vi "Menu_ItemName.vi"(7 "Ctrl":string, 8 "error in (no error)":errorcluster, 10 "DB Ref":T1, 11 "String":string) -> (0 "error out":errorcluster)   [LabVIEW 2017, in "tagdb-RefMgr Operations.lvlib"]
uses:
  tagdb-RefMgr Operations.lvlib
  <userlib>/_NEVSTOP/TagDB/Typedef/TagDB.ctl
  00d0da00-135c-4b50-b029-f1f1f0d03544.vi
  3fef5895-5f1b-4d45-a284-c279625095f7.vi
  4c542a80-f847-4821-836c-1c9f0a826a9d.vi
  00d0da00-135c-4b50-b029-f1f1f0d03544.vi/1b47866c-8e2d-43a7-815f-8cf18635e5a1.vi
  4c542a80-f847-4821-836c-1c9f0a826a9d.vi/1b47866c-8e2d-43a7-815f-8cf18635e5a1.vi
  <userlib>/_NEVSTOP/TagDB/_Support/Change Detector/TagDB dbChanged.vi
  <userlib>/_NEVSTOP/TagDB/_Support/Error/_Clear Errors.vi
  00d0da00-135c-4b50-b029-f1f1f0d03544.vi/1b47866c-8e2d-43a7-815f-8cf18635e5a1.vi/29b2ea6d-6d7f-4e4a-ad31-a5cb760462c7.vi
  <userlib>/_NEVSTOP/TagDB/API/TagDB-Status.vi
  4c542a80-f847-4821-836c-1c9f0a826a9d.vi/1b47866c-8e2d-43a7-815f-8cf18635e5a1.vi/29b2ea6d-6d7f-4e4a-ad31-a5cb760462c7.vi
  <userlib>/_NEVSTOP/TagDB/_Support/Change Detector/TagDB ChangeFlag.vi
  <userlib>/_NEVSTOP/TagDB/_Support/DataAccess/_NameCacher.vi
  <userlib>/_NEVSTOP/TagDB/_Support/Error/_[error50002]Invalid DataType.vi
  <userlib>/_NEVSTOP/TagDB/_Support/Error/_[error50000]Invalid DB REF.vi
  <userlib>/_NEVSTOP/TagDB/_Support/DataAccess/TagDB Ref to DVR.vi
  <userlib>/_NEVSTOP/TagDB/_Support/URL/TRIM-BOTH-SPACE.vi
  <userlib>/_NEVSTOP/TagDB/_Support/Error/_Build Error Cluster.vi
  <userlib>/_NEVSTOP/TagDB/TagDB.lvlib
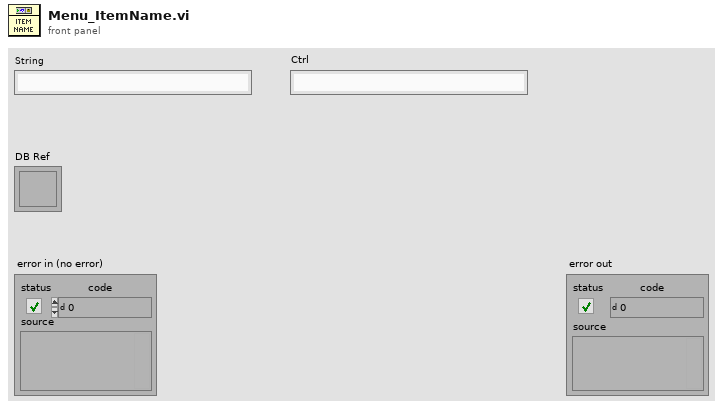
[diagram p1: front panel]
types:
  T1 = typedef "TagDB.lvlib/TagDB.ctl" = refnum<k1>
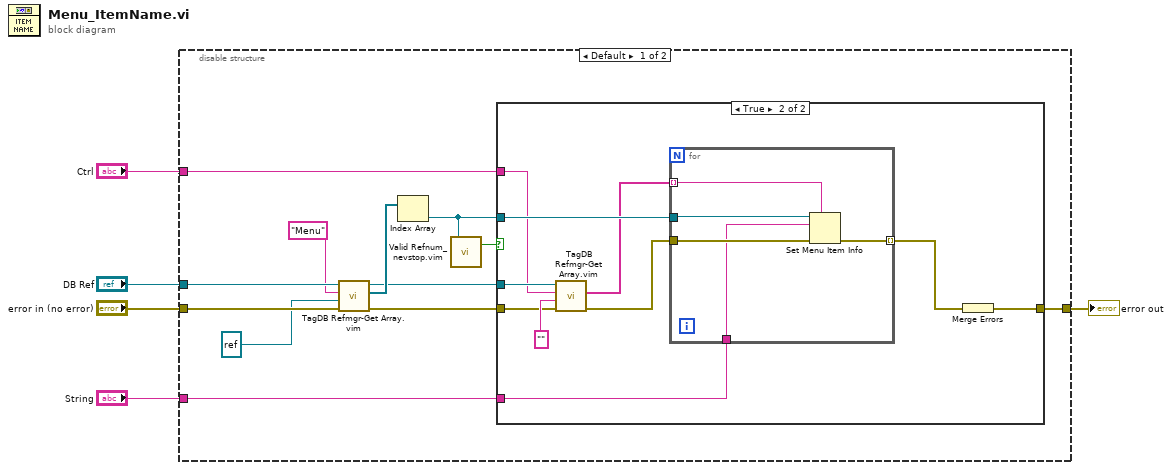
[diagram p0: block diagram]
diagram:
  n1 = disable-structure shown="Default" {
    disable-tunnel: "error in (no error)" -> [w17 w34]
    disable-tunnel: "DB Ref" -> [w16 _]
    disable-tunnel: "Ctrl" -> [w10 _]
    disable-tunnel: [w9 w34] -> w2
    disable-tunnel: "String" -> [w6 _]
    frame condition #0 (active) {
      n2 = call "TagDB Refmgr-Get Array.vim"("error in (no error)"=w17, "Type"=refnum<k9> refnum ("menu reference"), "RegExp"="Menu", "DB Ref"=w16) -> ("error out"=w8:errorcluster, "References"=w13:refnum<k9>[], "DB Ref(dup)"=w12:T1)  [unwired: 4 in, 1 out]
      n3 = Index Array(array=w13) -> (element=w11:refnum<k9>)  [unwired: 1 in]
      n4 = call "Valid Refnum_nevstop.vim"("number/path/refnum"=w11) -> ("Valid Number/Path/Refnum"=w7:bool)  [unwired: 2 in]
      n5 = case shown="True" w7 {
        tunnel: w12 -> [_ w28]
        tunnel: w11 -> [_ w27]
        tunnel: w10 -> [_ w25]
        tunnel: [w18 w22] -> w9
        tunnel: w8 -> [w18 w21]
        tunnel: w6 -> [_ w19]
        frame False {
        }
        frame True {
          n6 = call "TagDB Refmgr-Get Array.vim"("error in (no error)"=w21, "Type"="" ("RegExp"), "RegExp"=w25, "DB Ref"=w28) -> ("error out"=w20:errorcluster, "References"=w24:string[])  [unwired: 4 in, 2 out]
          n7 = for {
            tunnel: w27 -> [w33]
            tunnel: w24 -> [w32] mode=indexing
            tunnel: w20 -> [w31]
            tunnel: [w30] -> w23 mode=indexing
            tunnel: w19 -> [w29]
            n8 = Set Menu Item Info(7:w32, 8:w31, 10:w29, 11:w33) -> (0:w30:errorcluster)  [unwired: 3 in, 1 out]
          }
          n9 = Merge Errors(w23) -> (w22:errorcluster)
        }
      }
    }
    frame condition #1 {
    }
  }
  "error out" <- w2
